vi "sv_Check Data Valid [SRS].vi"(6 "critical damping factor":dbl=0.05 format="%.2f", 8 "error in (no error)":errorcluster, 10 "frequency range":T1={"low frequency [Hz]"=10.0, "high frequency [Hz]"=100.0, "frequencies / octave"=6} {"high frequency [Hz]" format="%.2f"; "low frequency [Hz]" format="%.2f"}, 11 "scaled signal [EU]":waveform(dbl)={"t0"=timestamp(0 s since 1904-01-01), "dt"=0.001, "Y"=[]}) -> (0 "error out":errorcluster, 2 "dup frequency range":T1={"low frequency [Hz]"=10.0, "high frequency [Hz]"=100.0, "frequencies / octave"=6} {"high frequency [Hz]" format="%.2f"; "low frequency [Hz]" format="%.2f"}, 3 "dup scaled signal [EU]":waveform(dbl)={"t0"=timestamp(0 s since 1904-01-01), "dt"=0.001, "Y"=[]}, 4 "dup critical damping":dbl=0.05 format="%.2f")   [LabVIEW 2017, in "SoundVib_Transient.lvlib"]
uses:
  <vilib>/addons/Sound and Vibration/svt_Transients/SoundVib_Transient.lvlib
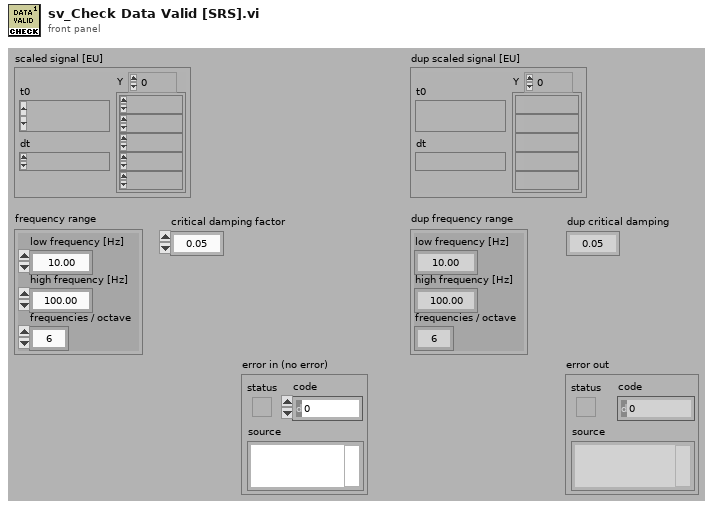
[diagram p1: front panel]
types:
  T1 = cluster{"low frequency [Hz]":dbl, "high frequency [Hz]":dbl, "frequencies / octave":i32}
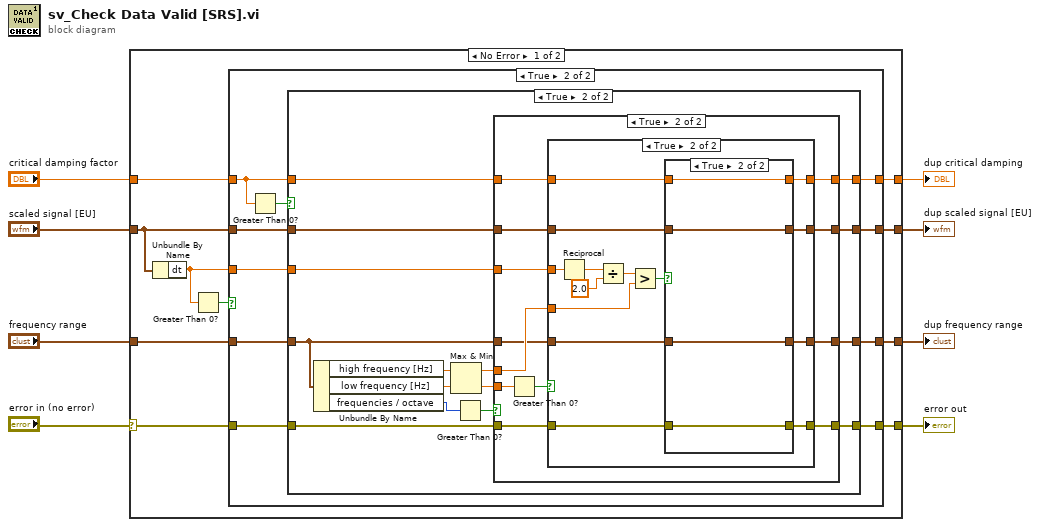
[diagram p0: block diagram]
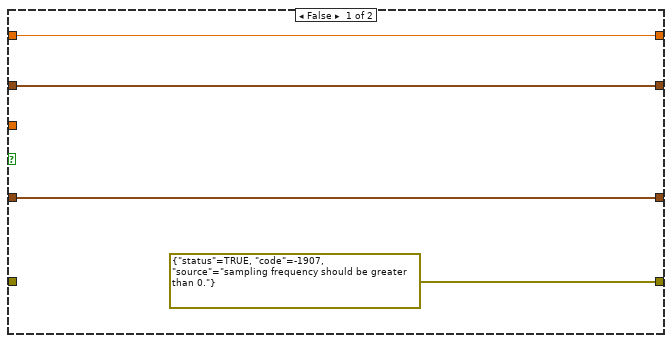
[diagram p2: hidden frame]
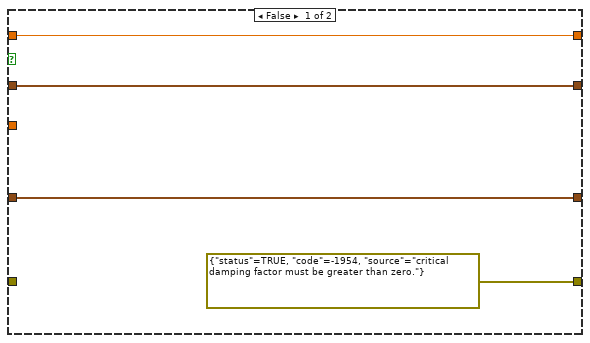
[diagram p3: hidden frame]
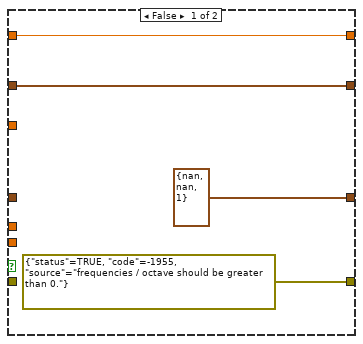
[diagram p4: hidden frame]
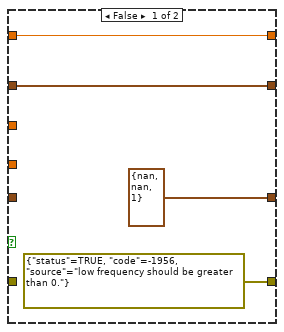
[diagram p5: hidden frame]
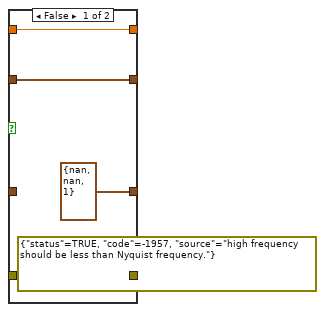
[diagram p6: hidden frame]
diagram:
  n1 = case shown="No Error" "error in (no error)" {
    selector: "error in (no error)" -> [w14 w97]
    tunnel: [w15 w97] -> w7
    tunnel: "scaled signal [EU]" -> [w12 w96]
    tunnel: "frequency range" -> [w17 w95]
    tunnel: [w13 w96] -> w4
    tunnel: [w11 w95] -> w3
    tunnel: "critical damping factor" -> [w10 w94]
    tunnel: [w9 w94] -> w1
    frame No Error {
      n2 = Unbundle By Name(w12) -> ("dt"=w16:dbl)
      n3 = Greater Than 0?(x=w16) -> (x > 0?=w18:bool)
      n4 = case shown="True" w18 {
        tunnel: w17 -> [w20 w26]
        tunnel: w16 -> [_ w32]
        tunnel: [errorcluster {"status"=TRUE, "code"=-1907, "source"="sampling frequency should be greater than 0."} ("error out") w31] -> w15
        tunnel: w14 -> [_ w30]
        tunnel: [w21 w29] -> w13
        tunnel: w12 -> [w21 w28]
        tunnel: [w20 w27] -> w11
        tunnel: w10 -> [w19 w24]
        tunnel: [w19 w23] -> w9
        frame False {
        }
        frame True {
          n5 = Greater Than 0?(x=w24) -> (x > 0?=w25:bool)
          n6 = case shown="True" w25 {
            tunnel: w32 -> [_ w46]
            tunnel: [errorcluster {"status"=TRUE, "code"=-1954, "source"="critical damping factor must be greater than zero."} ("error out") w44] -> w31
            tunnel: w30 -> [_ w43]
            tunnel: [w35 w42] -> w29
            tunnel: w28 -> [w35 w41]
            tunnel: [w34 w40] -> w27
            tunnel: w26 -> [w34 w39]
            tunnel: w24 -> [w33 w38]
            tunnel: [w33 w37] -> w23
            frame False {
            }
            frame True {
              n7 = Unbundle By Name(w39) -> ("high frequency [Hz]"=w49:dbl, "low frequency [Hz]"=w48:dbl, "frequencies / octave"=w51:i32)
              n8 = Max & Min(x=w49, y=w48) -> (max(x,y)=w45:dbl, min(x,y)=w47:dbl)
              n9 = Greater Than 0?(x=w51) -> (x > 0?=w50:bool)
              n10 = case shown="True" w50 {
                tunnel: w47 -> [_ w67]
                tunnel: w46 -> [_ w65]
                tunnel: w45 -> [_ w64]
                tunnel: [errorcluster {"status"=TRUE, "code"=-1955, "source"="frequencies / octave should be greater than 0."} ("error out") w63] -> w44
                tunnel: w43 -> [_ w62]
                tunnel: [w54 w61] -> w42
                tunnel: w41 -> [w54 w60]
                tunnel: [T1 {"low frequency [Hz]"=nan, "high frequency [Hz]"=nan, "frequencies / octave"=1} ("frequency range") w59] -> w40
                tunnel: w39 -> [_ w58]
                tunnel: w38 -> [w52 w57]
                tunnel: [w52 w56] -> w37
                frame False {
                }
                frame True {
                  n11 = Greater Than 0?(x=w67) -> (x > 0?=w66:bool)
                  n12 = case shown="True" w66 {
                    tunnel: w65 -> [_ w85]
                    tunnel: w64 -> [_ w81]
                    tunnel: [errorcluster {"status"=TRUE, "code"=-1956, "source"="low frequency should be greater than 0."} ("error out") w79] -> w63
                    tunnel: w62 -> [_ w78]
                    tunnel: [w70 w77] -> w61
                    tunnel: w60 -> [w70 w76]
                    tunnel: [T1 {"low frequency [Hz]"=nan, "high frequency [Hz]"=nan, "frequencies / octave"=1} ("frequency range") w75] -> w59
                    tunnel: w58 -> [_ w74]
                    tunnel: w57 -> [w68 w73]
                    tunnel: [w68 w72] -> w56
                    frame False {
                    }
                    frame True {
                      n13 = Reciprocal(x=w85) -> (1/x=w84:dbl)
                      n14 = Divide(x=w84, y=2.0) -> (x/y=w82:dbl)
                      n15 = Greater?(x=w82, y=w81) -> (0:w80:bool)
                      n16 = case shown="True" w80 {
                        tunnel: [errorcluster {"status"=TRUE, "code"=-1957, "source"="high frequency should be less than Nyquist frequency."} ("error out") w93] -> w79
                        tunnel: w78 -> [_ w93]
                        tunnel: [w88 w92] -> w77
                        tunnel: w76 -> [w88 w92]
                        tunnel: [T1 {"low frequency [Hz]"=nan, "high frequency [Hz]"=nan, "frequencies / octave"=1} ("frequency range") w91] -> w75
                        tunnel: w74 -> [_ w91]
                        tunnel: w73 -> [w86 w90]
                        tunnel: [w86 w90] -> w72
                        frame False {
                        }
                        frame True {
                        }
                      }
                    }
                  }
                }
              }
            }
          }
        }
      }
    }
    frame Error {
    }
  }
  "error out" <- w7
  "dup frequency range" <- w3
  "dup scaled signal [EU]" <- w4
  "dup critical damping" <- w1
